vi "TETRIX Motor Move_HT_myRIO.vi"(0 "Power (-100 to 100)\n0 = Stop/Brake\n-128 = Stop/Coast":i8(slide) scale=-100.0..100.0, 1 "Reverse? : T or F":bool, 2 "Control Mode":string(combo)="Power Only", 4 "Encoder Target: 360 = 1 motor shaft revolution":i32, 5 "Controller Daisy Chain Position: 1 - 4":u8=1 min=1 max=4, 6 "Select Channel":string(combo)="Motor 1", 7 "error in (no error)":errorcluster) -> (3 "error out":errorcluster)   [LabVIEW 2013]
uses:
  <vilib>/myRIO/Instrument Drivers/Onboard IO/I2C/vis/Smart Open.vi
  <vilib>/myRIO/Instrument Drivers/Onboard IO/I2C/vis/Configure.vi
  <vilib>/myRIO/Instrument Drivers/Onboard IO/I2C/vis/Write.vi
  <vilib>/myRIO/Instrument Drivers/Onboard IO/I2C/vis/Open.vi
  <vilib>/myRIO/Common/Instrument Driver Framework/myRIO v1.0/I2C/vis/myRIO v1.1 Open I2C.vi
  <vilib>/myRIO/Common/Instrument Driver Framework/Utilities/vis/Validate Channels.vi
  <vilib>/myRIO/Common/Instrument Driver Framework/myRIO v1.0/I2C/vis/myRIO v1.0 Reserve I2C.vi
  <vilib>/myRIO/Common/Instrument Driver Framework/myRIO v1.0/I2C/vis/myRIO v1.0 Build MUX Configuration I2C.vi
  <vilib>/myRIO/Common/Instrument Driver Framework/myRIO v1.0/Resource Manager/vis/myRIO v1.0 Reserve Channel List.vi
  <vilib>/myRIO/Common/Instrument Driver Framework/myRIO v1.0/Resource Manager/vis/myRIO v1.0 Create Configuration List.vi
  <vilib>/myRIO/Common/Instrument Driver Framework/myRIO v1.0/Resource Manager/vis/myRIO v1.0 Reserve Channel.vi
  <vilib>/myRIO/Common/Instrument Driver Framework/myRIO v1.0/Resource Manager/vis/myRIO v1.0 Unreserve Channel.vi
  <vilib>/myRIO/Common/Instrument Driver Framework/myRIO v1.0/Resource Manager/vis/myRIO v1.0 Build Mutex Name.vi
  <vilib>/myRIO/Common/Instrument Driver Framework/myRIO v1.0/myRIO v1.1 Open.vi
  <vilib>/Utility/VariantDataType/GetNumericInfo.vi
  <vilib>/Utility/error.llb/Error Cluster From Error Code.vi
  <vilib>/myRIO/Common/Instrument Driver Framework/Utilities/vis/IO Manager.vi
  <vilib>/myRIO/Common/Instrument Driver Framework/Utilities/vis/Configuration Manager.vi
  <vilib>/myRIO/Common/Instrument Driver Framework/myRIO v1.0/Resource Manager/vis/myRIO v1.0 Configure IO.vi
  <vilib>/myRIO/Common/Instrument Driver Framework/myRIO v1.0/myRIO v1.0 Close.vi
  <vilib>/myRIO/Common/Instrument Driver Framework/myRIO v1.0/I2C/vis/myRIO v1.0 Configure I2C.vi
  <vilib>/myRIO/Common/Instrument Driver Framework/myRIO v1.0/I2C/vis/myRIO v1.0 Write I2C.vi
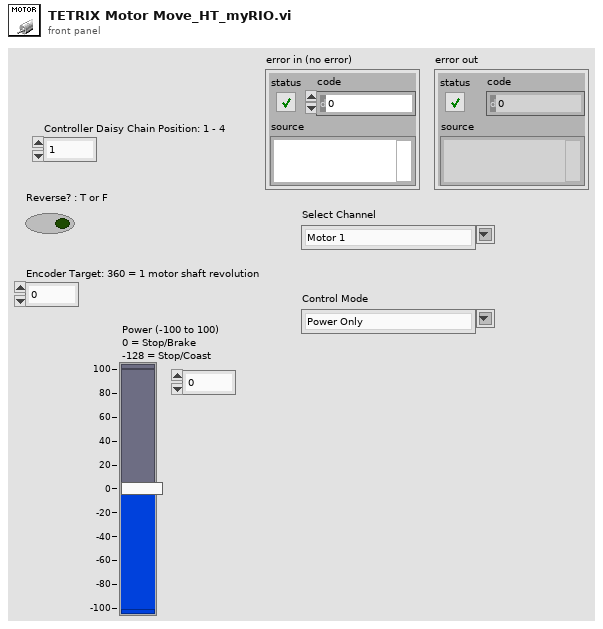
[diagram p1: front panel]
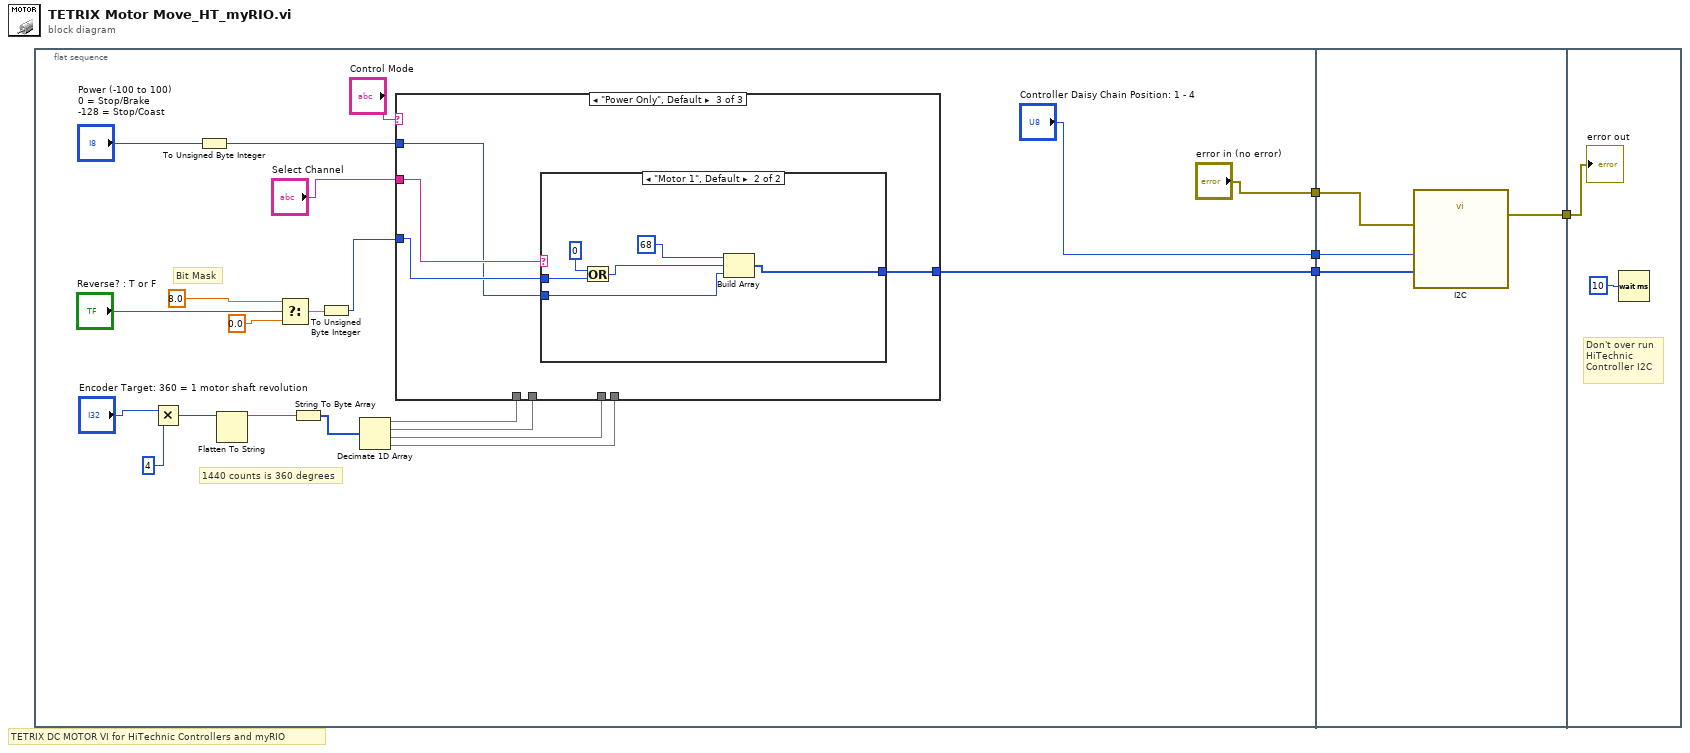
[diagram p0: block diagram]
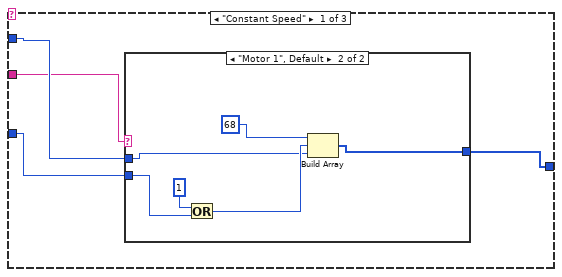
[diagram p2: hidden frame]
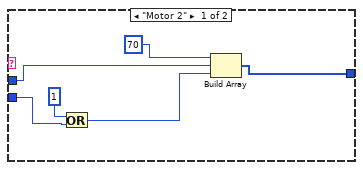
[diagram p3: hidden frame]
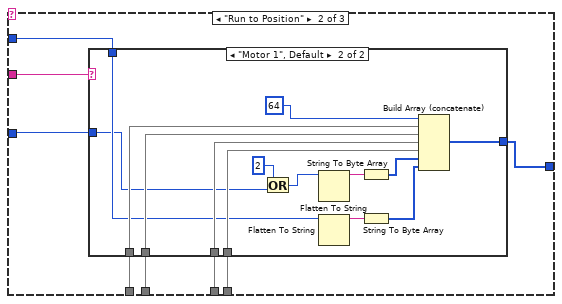
[diagram p4: hidden frame]
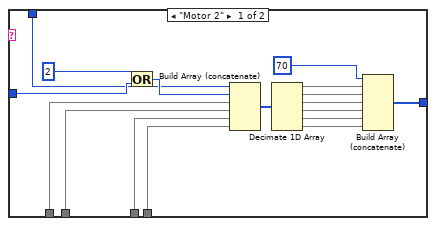
[diagram p5: hidden frame]
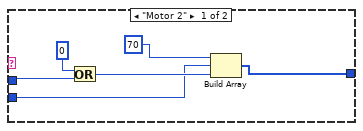
[diagram p6: hidden frame]
diagram:
  # "TETRIX DC MOTOR VI for HiTechnic Controllers and myRIO"
  n1 = flat-sequence {
    tunnel: ["Controller Daisy Chain Position: 1 - 4"] -> w4
    tunnel: [w14] -> w3
    tunnel: ["error in (no error)"] -> w2
    tunnel: w4 -> [w100]
    tunnel: w3 -> [w99]
    tunnel: w2 -> [w98]
    tunnel: [w97] -> w1
    tunnel: w1 -> [w101]
    frame #0 {
      # "1440 counts is 360 degrees"
      # "Bit Mask"
      n2 = Multiply(x="Encoder Target: 360 = 1 motor shaft revolution", y=4) -> (x*y=w6:i32)
      n3 = To Unsigned Byte Integer(number="Power (-100 to 100)\n0 = Stop/Brake\n-128 = Stop/Coast") -> (unsigned 8bit integer=w16:u8)
      n4 = Flatten To String(anything=w6) -> (data string=w25:string)  [unwired: 3 in, 2 out]
      n5 = Select(t=8.0, s="Reverse? : T or F", f=0.0) -> (s? t:f=w21:dbl)
      n6 = String To Byte Array(string=w25) -> (unsigned byte array=w13:u8[])
      n7 = To Unsigned Byte Integer(number=w21) -> (unsigned 8bit integer=w17:u8)
      n8 = Decimate 1D Array(w13) -> (w12:u8[], w11:u8[], w10:u8[], w9:u8[])
      n9 = case shown="\"Power Only\", Default" "Control Mode" {
        tunnel: "Select Channel" -> [w26 w49 w84]
        tunnel: w17 -> [w28 w48 w83]
        tunnel: w16 -> [w29 w47 w82]
        tunnel: [w27 w46 w81] -> w14
        tunnel: w12 -> [_ w45 _]
        tunnel: w11 -> [_ w44 _]
        tunnel: w10 -> [_ w43 _]
        tunnel: w9 -> [_ w42 _]
        frame "Constant Speed" {
          n10 = case shown="\"Motor 1\", Default" w26 {
            tunnel: w29 -> [w31 w36]
            tunnel: w28 -> [w32 w38]
            tunnel: [w33 w39] -> w27
            frame "Motor 2" {
              n11 = Or(x=u8 1, y=w32) -> (x .or. y?=w30:u8)
              n12 = Build Array(u8 70, w31, w30) -> (w33:u8[])
            }
            frame "Motor 1", Default {
              n13 = Or(x=u8 1, y=w38) -> (x .or. y?=w37:u8)
              n14 = Build Array(u8 68, w37, w36) -> (w39:u8[])
            }
          }
        }
        frame "Run to Position" {
          n15 = case shown="\"Motor 1\", Default" w49 {
            tunnel: w48 -> [w56 w67]
            tunnel: w47 -> [w55 w70]
            tunnel: [w54 w78] -> w46
            tunnel: w45 -> [w53 w71]
            tunnel: w44 -> [w52 w72]
            tunnel: w43 -> [w51 w73]
            tunnel: w42 -> [w50 w74]
            frame "Motor 2" {
              n16 = Or(x=u8 2, y=w56) -> (x .or. y?=w57:u8)
              n17 = Build Array (concatenate)(w55, w57, w53, w52, w51, w50) -> (w66:u8[])
              n18 = Decimate 1D Array(w66) -> (w60:u8[], w61:u8[], w62:u8[], w63:u8[], w64:u8[], w65:u8[])
              n19 = Build Array (concatenate)(u8 70, w60, w61, w62, w63, w64, w65) -> (w54:u8[])
            }
            frame "Motor 1", Default {
              n20 = Or(x=u8 2, y=w67) -> (x .or. y?=w68:u8)
              n21 = Flatten To String(anything=w68) -> (data string=w79:string)  [unwired: 3 in, 2 out]
              n22 = Flatten To String(anything=w70) -> (data string=w80:string)  [unwired: 3 in, 2 out]
              n23 = String To Byte Array(string=w79) -> (unsigned byte array=w75:u8[])
              n24 = String To Byte Array(string=w80) -> (unsigned byte array=w76:u8[])
              n25 = Build Array (concatenate)(u8 64, w71, w72, w73, w74, w75, w76) -> (w78:u8[])
            }
          }
        }
        frame "Power Only", Default {
          n26 = case shown="\"Motor 1\", Default" w84 {
            tunnel: w83 -> [w88 w94]
            tunnel: w82 -> [w85 w91]
            tunnel: [w87 w93] -> w81
            frame "Motor 2" {
              n27 = Or(x=u8 0, y=w88) -> (x .or. y?=w86:u8)
              n28 = Build Array(u8 70, w85, w86) -> (w87:u8[])
            }
            frame "Motor 1", Default {
              n29 = Or(x=u8 0, y=w94) -> (x .or. y?=w92:u8)
              n30 = Build Array(u8 68, w92, w91) -> (w93:u8[])
            }
          }
        }
      }
    }
    frame #1 {
      n31 = call "I2C"("Slave Address (7-bit)"=w100, "Bytes to Write"=w99, "error in (no error)"=w98) -> ("error out"=w97:errorcluster)  [unwired: 24 in]
    }
    frame #2 {
      # "Don't over run\nHiTechnic\nController I2C"
      n32 = Wait (ms)(milliseconds to wait=u32 10) -> ()  [unwired: 1 out]
      "error out" <- w101
    }
  }
